vi "Pre Launch Init.vi"(11 "MonitoredMediator in":refnum<class "MonitoredMediator.lvclass">) -> (0 "error out":errorcluster, 3 "MonitoredMediator out":refnum<class "MonitoredMediator.lvclass">)   [LabVIEW 2017, in "MonitoredMediator.lvlib" / "MonitoredMediator.lvclass"]
doc: "(<B>Filename</B>: Actor Framework.lvlib:Actor.lvclass:Pre Launch Init.vi)\n\nDefines behavior that occurs after the Launch Nested Actor method is invoked but before the actor's Actor Core method begins running.\n\nBy default, this method does nothing. A descendant class may override it to define behavior."
uses:
  <vilib>/gpm_packages/@cs/mva-core/Source/MonitoredMediator/MonitoredMediator/MonitoredMediator.lvclass
  C:/Program Files/National Instruments/LabVIEW 2017/vi.lib/ActorFramework/Actor/Actor.lvclass
  <vilib>/ActorFramework/Actor/Actor.lvclass/Actor.ctl
  <vilib>/ActorFramework/Message Enqueuer/Message Enqueuer.lvclass/Message Enqueuer.ctl
  <vilib>/gpm_packages/@cs/mva-core/Source/MonitoredMediator/MonitoredMediator/MonitoredMediator.lvclass/MonitoredMediator.ctl
  <vilib>/gpm_packages/@cs/mva-core/Source/MonitoredMediator/IBusMonitor/IBusMonitor.lvclass
  <vilib>/ActorFramework/Message Enqueuer/Message Priority.ctl
  <vilib>/gpm_packages/@cs/mva-core/Source/MonitoredMediator/MonitoredMediator Messages/Attach Bus Monitor Msg/Attach Bus Monitor Msg.lvclass/Attach Bus Monitor Msg.ctl
  <vilib>/ActorFramework/Message Enqueuer/Init from Existing Queue.vi
  <vilib>/ActorFramework/Message Enqueuer/Enqueue.vi
  <vilib>/gpm_packages/@cs/mva-core/Source/MonitoredMediator/MonitoredMediator Messages/Attach Bus Monitor Msg/Attach Bus Monitor Msg.lvclass
  C:/Program Files/National Instruments/LabVIEW 2017/vi.lib/ActorFramework/Message/Message.lvclass
  <vilib>/ActorFramework/Message Priority Queue/Priority Enqueue.vi
  <vilib>/ActorFramework/Message Enqueuer/Message Enqueuer.lvclass
  <vilib>/gpm_packages/@cs/mva-core/Source/Mediator/Mediator/Mediator.lvclass
  <vilib>/ActorFramework/Actor/Actor.lvclass
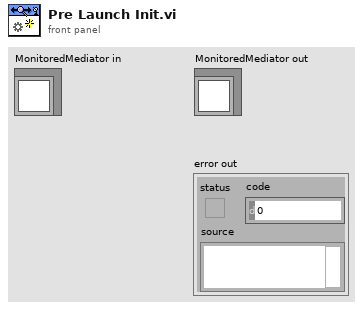
[diagram p1: front panel]
types:
  T1 = typedef "Actor Framework.lvlib/Message Enqueuer.lvclass/Message Priority.ctl" = enum16{"Low", "Normal", "High"}
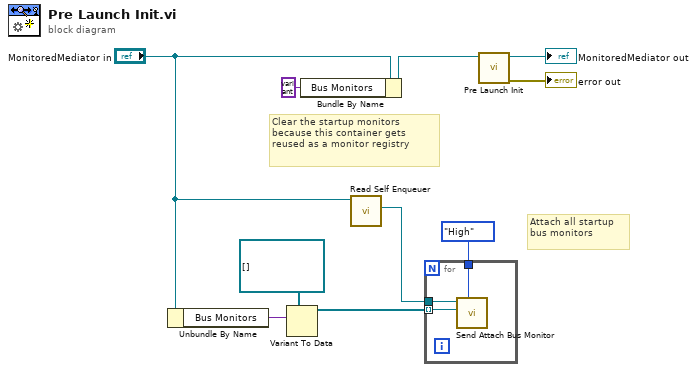
[diagram p0: block diagram]
diagram:
  # "Attach all startup\nbus monitors"
  # "Clear the startup monitors\nbecause this container gets\nreused as a monitor registry"
  n1 = Unbundle By Name("MonitoredMediator in") -> ("Bus Monitors"=w8:variant)
  n2 = Variant To Data(type=refnum<class "IBusMonitor.lvclass">[] [] ("Array"), Variant=w8) -> (data=w2:refnum<class "IBusMonitor.lvclass">[])  [unwired: 1 in, 1 out]
  n3 = Bundle By Name(cluster="MonitoredMediator in", "Bus Monitors"=variant) -> (w4:refnum<class "MonitoredMediator.lvclass">)
  n4 = call <vilib>:"Read Self Enqueuer.vi"("Actor"="MonitoredMediator in") -> ("Self Enqueuer"=w5:refnum<class "Message Enqueuer.lvclass">)  [unwired: 10 in]
  n5 = for {
    tunnel: w5 -> [w13]
    tunnel: w2 -> [w12] mode=indexing
    tunnel: Message_Priority."High" ("Message Priority (Normal)") -> [w11]
    n6 = call <vilib>:"Send Attach Bus Monitor.vi"("Message Priority (Normal)"=w11, "BusMonitor"=w12, "Message Enqueuer"=w13) -> ()  [unwired: 7 in, 2 out]
  }
  n7 = call-parent "Pre Launch Init.vi"("Mediator in"=w4) -> ("error out"=→"error out":errorcluster, "Mediator out"=→"MonitoredMediator out":refnum<class "MonitoredMediator.lvclass">)  [unwired: 9 in]
